vi "rotmrev.vi"(6 "reverse":bool, 7 "angle[rad]":dbl, 8 "x":dbl[](array[numeric]), 9 "y":dbl[](array[numeric]), 10 "x0":dbl, 11 "y0":dbl) -> (2 "y":dbl[](array[numeric]), 3 "x":dbl[](array[numeric]))   [LabVIEW 2015]
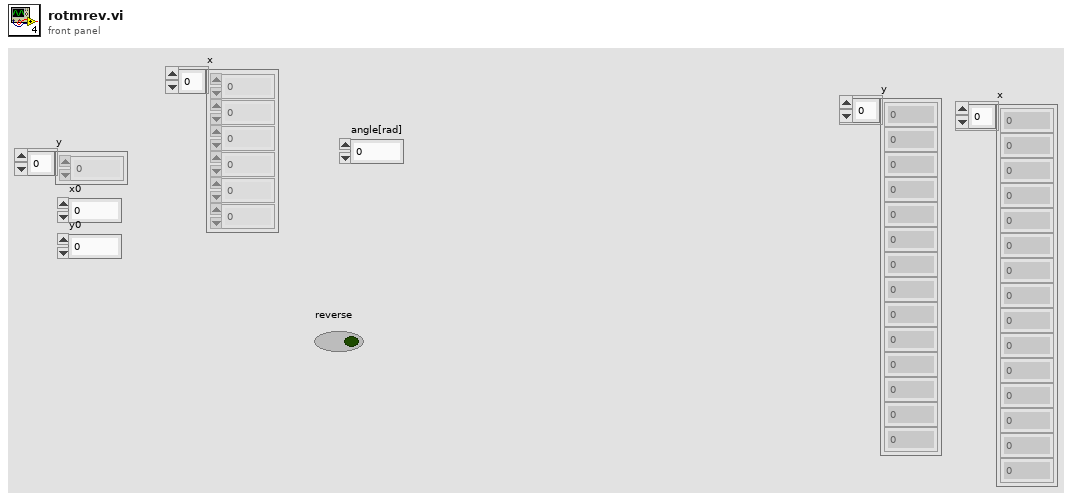
[diagram p1: front panel]
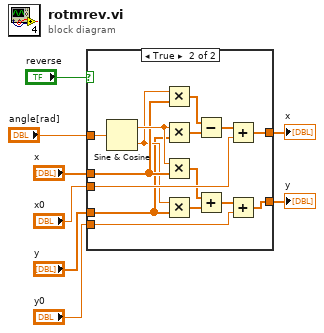
[diagram p0: block diagram]
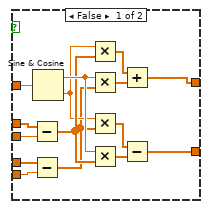
[diagram p2: hidden frame]
diagram:
  n1 = case shown="True" "reverse" {
    tunnel: "angle[rad]" -> [w19 w38]
    tunnel: "x" -> [w23 w32]
    tunnel: "x0" -> [w22 w34]
    tunnel: "y0" -> [w20 w26]
    tunnel: "y" -> [w21 w30]
    tunnel: [w10 w25] -> w3
    tunnel: [w9 w24] -> w1
    frame False {
      n2 = Subtract(x=w23, y=w22) -> (x-y=w15:dbl[])
      n3 = Subtract(x=w21, y=w20) -> (x-y=w13:dbl[])
      n4 = Sine & Cosine(0:w19) -> (1:w16:dbl, 2:w14:dbl)
      n5 = Multiply(x=w14, y=w15) -> (x*y=w18:dbl[])
      n6 = Multiply(x=w16, y=w13) -> (x*y=w17:dbl[])
      n7 = Multiply(x=w14, y=w13) -> (x*y=w12:dbl[])
      n8 = Multiply(x=w16, y=w15) -> (x*y=w11:dbl[])
      n9 = Add(x=w18, y=w17) -> (x+y=w10:dbl[])
      n10 = Subtract(x=w12, y=w11) -> (x-y=w9:dbl[])
    }
    frame True {
      n11 = Sine & Cosine(0:w38) -> (1:w33:dbl, 2:w31:dbl)
      n12 = Multiply(x=w31, y=w32) -> (x*y=w37:dbl[])
      n13 = Multiply(x=w33, y=w30) -> (x*y=w36:dbl[])
      n14 = Multiply(x=w33, y=w32) -> (x*y=w29:dbl[])
      n15 = Multiply(x=w31, y=w30) -> (x*y=w28:dbl[])
      n16 = Subtract(x=w37, y=w36) -> (x-y=w35:dbl[])
      n17 = Add(x=w29, y=w28) -> (x+y=w27:dbl[])
      n18 = Add(x=w35, y=w34) -> (x+y=w25:dbl[])
      n19 = Add(x=w27, y=w26) -> (x+y=w24:dbl[])
    }
  }
  "x" <- w3
  "y" <- w1
